vi "Table-Set header string.vi"(8 "error in (no error)":errorcluster, 9 "Row/Column":enum16{"Row header", "Column header"}(ring), 10 "Column header string":string caption="Header string", 11 "Table":refnum<vi>) -> (0 "error out":errorcluster, 3 "Table out":refnum<vi>)   [LabVIEW 2017]
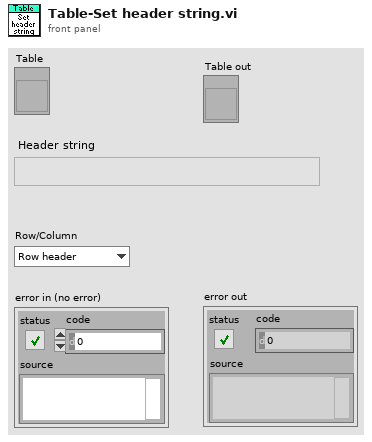
[diagram p1: front panel]
types:
  T1 = typedef "LVRowAndColumnTypeDef.ctl" = cluster{"Row":i32, "Column":i32}
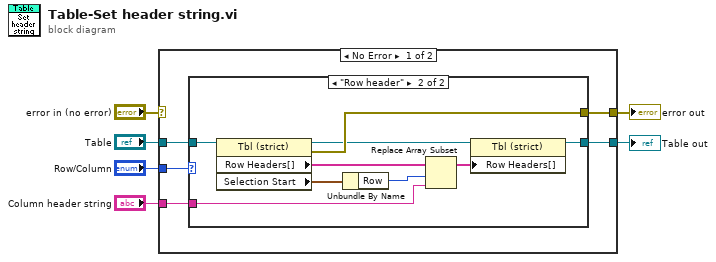
[diagram p0: block diagram]
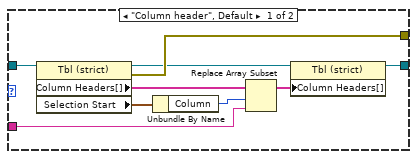
[diagram p2: hidden frame]
diagram:
  n1 = case shown="No Error" "error in (no error)" {
    selector: "error in (no error)" -> [_ w31]
    tunnel: "Table" -> [w11 w30]
    tunnel: [w10 w30] -> w5
    tunnel: "Row/Column" -> [w9 _]
    tunnel: [w8 w31] -> w2
    tunnel: "Column header string" -> [w7 _]
    frame No Error {
      n2 = case shown="\"Row header\"" w9 {
        tunnel: w11 -> [w20 w29]
        tunnel: [w14 w23] -> w10
        tunnel: [w16 w25] -> w8
        tunnel: w7 -> [w12 w21]
        frame "Column header", Default {
          n3 = property class="Tbl (strict)"(reference=w20) -> (reference out=w15:refnum<vi>, error out=w16:errorcluster, "Column Headers[]"=w18:string[], "Selection Start"=w19:T1)  [unwired: 1 in]
          n4 = Unbundle By Name(w19) -> ("Column"=w17:i32)
          n5 = Replace Array Subset(array=w18, new element=w12, index=w17) -> (w13:string[])
          n6 = property class="Tbl (strict)"(reference=w15, "Column Headers[]"=w13) -> (reference out=w14:refnum<vi>)  [unwired: 1 in, 1 out]
        }
        frame "Row header" {
          n7 = property class="Tbl (strict)"(reference=w29) -> (reference out=w24:refnum<vi>, error out=w25:errorcluster, "Row Headers[]"=w27:string[], "Selection Start"=w28:T1)  [unwired: 1 in]
          n8 = Unbundle By Name(w28) -> ("Row"=w26:i32)
          n9 = Replace Array Subset(array=w27, new element=w21, index=w26) -> (w22:string[])
          n10 = property class="Tbl (strict)"(reference=w24, "Row Headers[]"=w22) -> (reference out=w23:refnum<vi>)  [unwired: 1 in, 1 out]
        }
      }
    }
    frame Error {
    }
  }
  "Table out" <- w5
  "error out" <- w2
